vi "PlayChords.vi"() -> (3 "timed out?":bool)   [LabVIEW 2016]
uses:
  <vilib>/Platform/TimedLoop/XDataNode/timing_clust.ctl
  <vilib>/Platform/TimedLoop/XDataNode/nitl_modes.ctl
  <vilib>/Platform/TimedLoop/XDataNode/wakeup.ctl
  <vilib>/sound2/lvsound2.llb/Sound Data Format.ctl
  <vilib>/sound2/lvsound2.llb/Sampling Mode.ctl
  <vilib>/sound2/lvsound2.llb/Sound Output Set Volume (Single).vi
  <vilib>/sound2/lvsound2.llb/Sound Output Write (DBL).vi
  <vilib>/express/express analysis/Spectral/Block/exnSpectralBlock spectral measurements power poly.vi
  <vilib>/express/express analysis/Spectral/Block/exnSpectralBlock spectral measurements power WFM.vi
  <vilib>/platform/TimedLoop/XDataNode/XDataNode.xnode
  <vilib>/express/express analysis/Spectral/XNode/ExpressSpectralMeasurementsBlockNode.xnode
  <vilib>/Platform/TimedLoop/XDataNode/XDNodeRunTimeDep.lvlib
panel:
  out "#Note DiatonicScale":u8
  out "fretPosition":dbl[](array[numeric])
  out "#StringsUsed in Chord":dbl
  out "Power Spectrum":cluster{"f0":dbl, "df":dbl, "magnitude":dbl[]}(graph)
  in  "?":bool
  in  "Volume 2":dbl(knob)=35.90378919003022 scale=20.0..100.0
  in  "strumming rate (in ms)":dbl=10.0
  in  "Upstrum ?":bool
  # "0, 1, 8 -> C mojor chord\n2 -> D major chord\n3 -> E major chord\n4 -> F major chord\n5 -> G major chord\n6 -> A major chord\n7 -> B mojor chord"
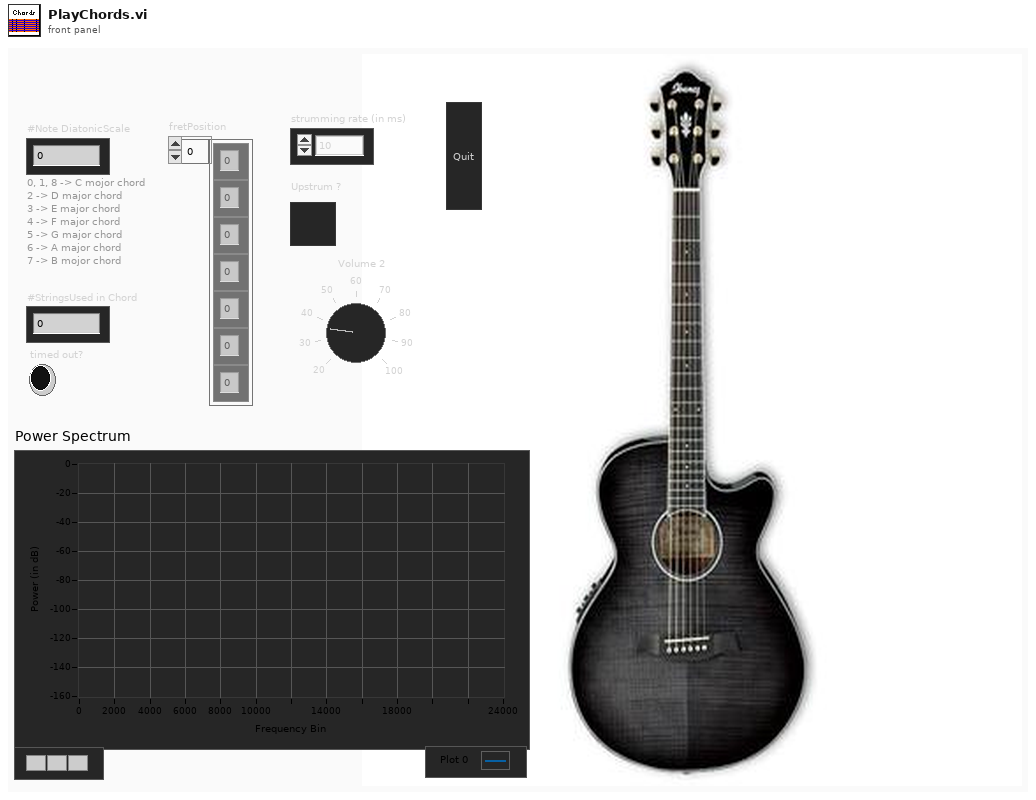
[diagram p1: front panel]
types:
  T1 = typedef "XDNodeRunTimeDep.lvlib/timing_clust.ctl" = cluster{"Expected End [f-1]":u64, "Actual End [f-1]":u64, "Finished Late? [f-1]":bool, "Expected End [i-1]":u64, "Actual End [i-1]":u64, "Finished Late? [i-1]":bool, "Expected Start [i]":u64, "Actual Start [i]":u64, "Expected Start [f]":u64, "Actual Start [f]":u64, "Source Name":string, "Structure Name":string, "Period":i64, "Deadline":i64, "Offset":i64, "Start":i64, "Priority":i32, "Timeout":i32, "Mode":T2, "Wakeup Reason":T3, "Error":errorcluster, "Source Type":string, "Secondary Source Type":string, "Global End Time":u64, "Global Start Time":u64, "Frame Duration":u64, "Iteration Duration":u64, "Assigned CPU":i32, "I/O Scan Engine Mode":u32}
  T2 = typedef "XDNodeRunTimeDep.lvlib/nitl_modes.ctl" = enum32{"No Change", "Process missed periods, maintain original phase", "Discard missed periods, maintain original phase", "Process missed periods, ignore original phase", "Discard missed periods, ignore original phase"}
  T3 = typedef "XDNodeRunTimeDep.lvlib/wakeup.ctl" = enum32{"Normal", "Aborted", "Asynchronous wakeup", "Timing source error", "Timed loop error", "Timeout"}
  T4 = typedef "Sound Data Format.ctl" = cluster{"sample rate (S/s)":dbl, "number of channels":i32, "bits per sample":i32}
  T5 = cluster{"averaging mode":u16, "weighting mode":u16, "number of averages":u32}
  T6 = cluster{"dB On (F)":bool, "unwrap phase (F)":bool, "convert to degree (F)":bool}
  T7 = typedef "Sampling Mode.ctl" = i32
  T8 = typedef "Sound Output Task ID.ctl" = u32
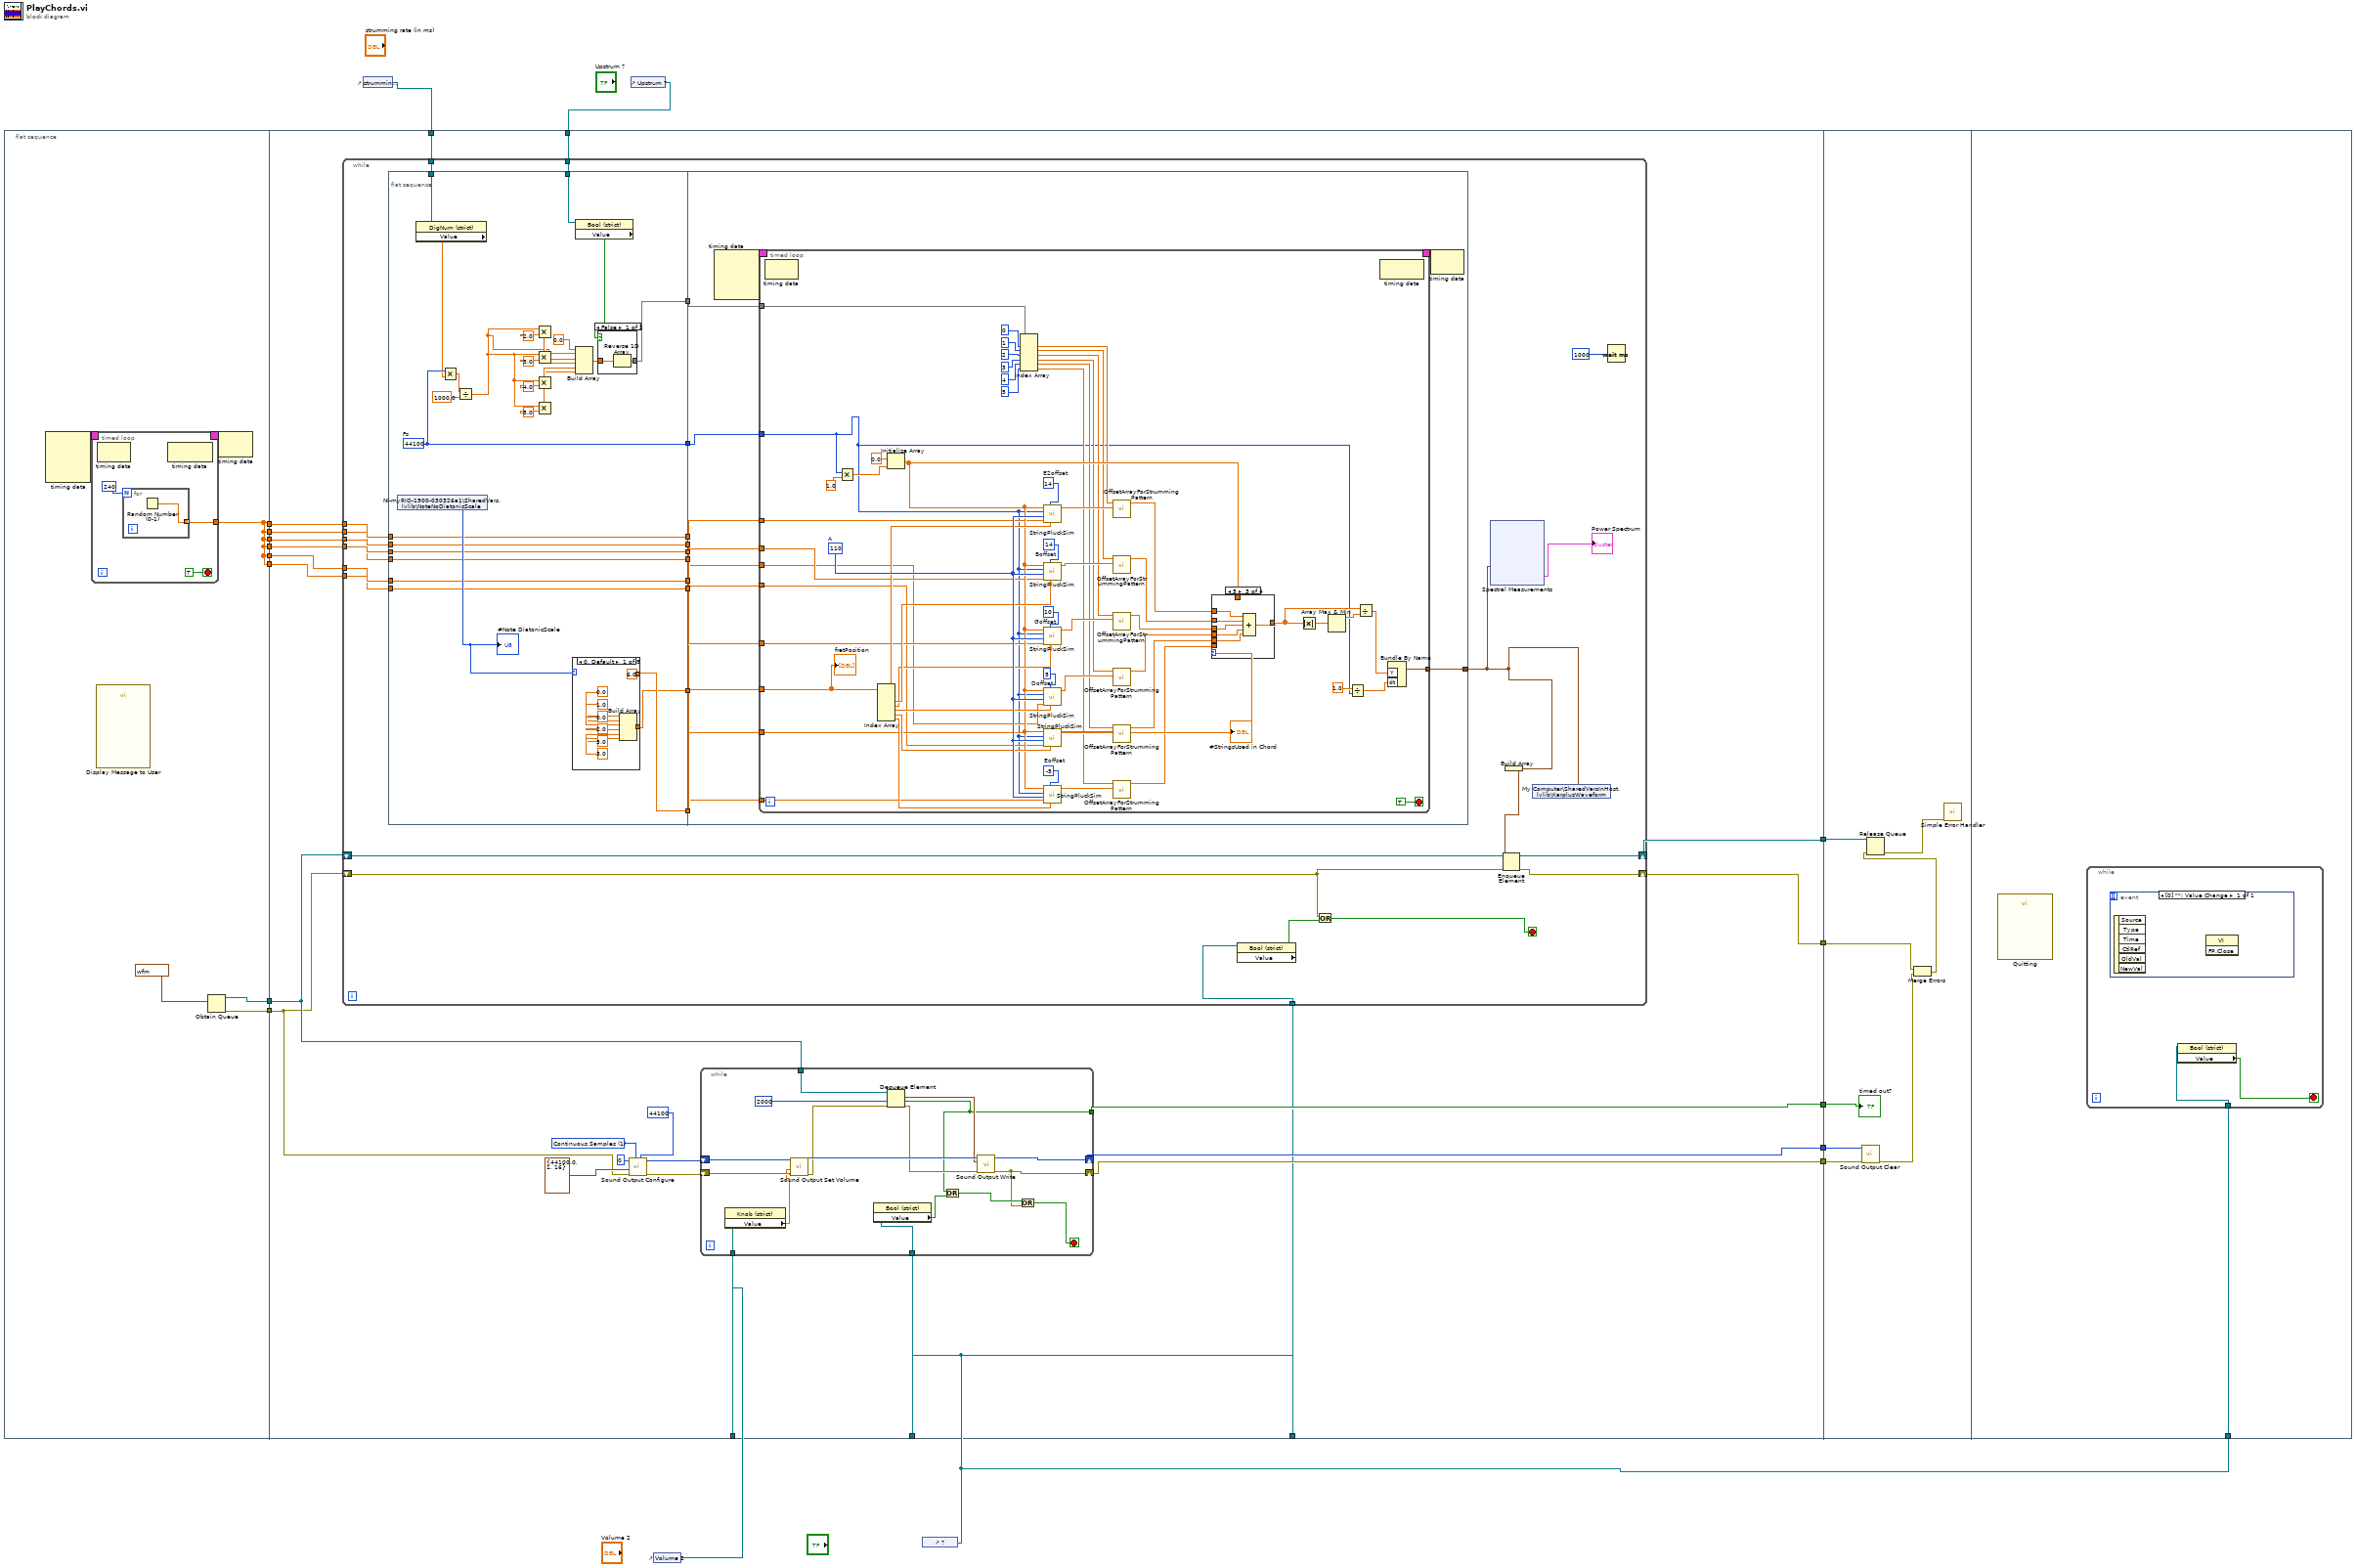
[diagram p0: block diagram]
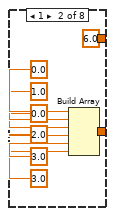
[diagram p3: hidden frame]
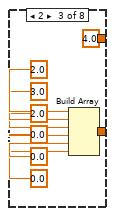
[diagram p4: hidden frame]
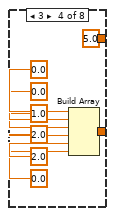
[diagram p5: hidden frame]
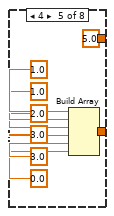
[diagram p6: hidden frame]
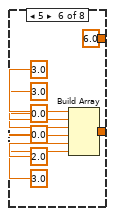
[diagram p7: hidden frame]
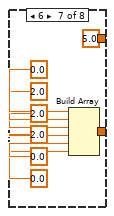
[diagram p8: hidden frame]
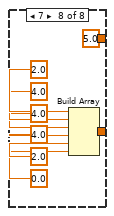
[diagram p9: hidden frame]
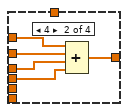
[diagram p11: hidden frame]
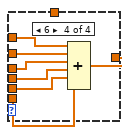
[diagram p12: hidden frame]
diagram:
  n1 = flat-sequence {
    tunnel: [w20] -> w17
    tunnel: [w22] -> w16
    tunnel: [w21] -> w15
    tunnel: [w20] -> w14
    tunnel: [w20] -> w13
    tunnel: [w20] -> w12
    tunnel: [w20] -> w11
    tunnel: [w20] -> w10
    tunnel: w17 -> [w47]
    tunnel: w16 -> [w49]
    tunnel: w15 -> [w48]
    tunnel: w14 -> [w46]
    tunnel: w13 -> [w45]
    tunnel: w12 -> [w44]
    tunnel: w11 -> [w43]
    tunnel: w10 -> [w42]
    tunnel: w3 -> [w41]
    tunnel: w4 -> [w40]
    tunnel: w2 -> [w39]
    tunnel: [w38] -> w9
    tunnel: [w37] -> w8
    tunnel: [w35] -> w7
    tunnel: [w36] -> w6
    tunnel: [w34] -> w5
    tunnel: w1 -> [w33]
    tunnel: w1 -> [w32]
    tunnel: w9 -> [w305]
    tunnel: w8 -> [w304]
    tunnel: w7 -> [w303]
    tunnel: w6 -> [w302]
    tunnel: w5 -> [w301]
    tunnel: w1 -> [w308]
    frame #0 {
      n2 = node-c288() -> (w19:T1)  [unwired: 4 in]
      n3 = timed-loop {
        timing: w19 -> [_]
        timing-out: [_] -> w18
        tunnel: [w25] -> w20
        stop <- TRUE stop-if-true
        n4 = node-c288() -> ()  [unwired: 1 in, 1 out]
        n5 = for {
          N: 240 -> [_]
          tunnel: [w27] -> w25 mode=indexing
          n6 = Random Number (0-1)() -> (number: 0 to 1=w27:dbl)
        }
        n7 = node-c288() -> ()  [unwired: 1 in, 1 out]
      }
      n8 = call "Display Message to User"() -> ()  [unwired: 10 in, 2 out]
      n9 = Obtain Queue(element data type=waveform(dbl)[] [{"t0"=timestamp(3482746353.0334034 s since 1904-01-01), "dt"=4.5351473922902495e-05, "Y"=array[5000 elements]}, {"t0"=timestamp(3482746353.0334034 s since 1904-01-01), "dt"=4.5351473922902495e-05, "Y"=array[5000 elements]}] ("Generated Sound")) -> (queue out=w22:refnum<queue>, error out=w21:errorcluster)  [unwired: 4 in, 1 out]
      n10 = node-c288(w18) -> ()  [unwired: 1 out]
    }
    frame #1 {
      w53 = T7 1 items=["Finite Samples", "Continuous Samples"] ("sample mode")
      n11 = while {
        shift-right: [w82] -> w38
        shift-left: w49 -> [w84]
        shift-right: [w83] -> w37
        shift-left: w48 -> [w80]
        tunnel: w47 -> [w75]
        tunnel: w46 -> [w73]
        tunnel: w45 -> [w71]
        tunnel: w44 -> [w69]
        tunnel: w43 -> [w67]
        tunnel: w42 -> [w65]
        tunnel: w41 -> [w62]
        tunnel: w40 -> [w61]
        tunnel: w32 -> [w59]
        stop <- w81 stop-if-true
        n12 = flat-sequence {
          tunnel: [w120] -> w78
          tunnel: [w119] -> w77
          tunnel: [w118] -> w76
          tunnel: w75 -> [w118]
          tunnel: [w117] -> w74
          tunnel: w73 -> [w117]
          tunnel: [w116] -> w72
          tunnel: w71 -> [w116]
          tunnel: [w115] -> w70
          tunnel: w69 -> [w115]
          tunnel: [w114] -> w68
          tunnel: w67 -> [w114]
          tunnel: [w113] -> w66
          tunnel: w65 -> [w113]
          tunnel: [w102] -> w64
          tunnel: [w101] -> w63
          tunnel: w62 -> [w97]
          tunnel: w61 -> [w95]
          tunnel: [w201] -> w56
          tunnel: w78 -> [w200]
          tunnel: w77 -> [w199]
          tunnel: w76 -> [w198]
          tunnel: w74 -> [w197]
          tunnel: w72 -> [w196]
          tunnel: w70 -> [w195]
          tunnel: w68 -> [w194]
          tunnel: w66 -> [w193]
          tunnel: w64 -> [w192]
          tunnel: w63 -> [w191]
          frame #0 {
            w101 = 44100  # Fs
            n13 = shared-variable "NI-myRIO-1900-030326a1\\SharedVars.lvlib\\NoteNoDiatonicScale"() -> (w121:u8)  [unwired: 1 in, 1 out]
            "#Note DiatonicScale" <- w121
            n14 = property class="DigNum (strict)"(reference=w97) -> ("Value"=w96:dbl)  [unwired: 1 in, 2 out]
            n15 = Multiply(x=w101, y=w96) -> (x*y=w100:dbl)
            n16 = Divide(x=w100, y=1000.0) -> (x/y=w98:dbl)
            n17 = Multiply(x=w98, y=2.0) -> (x*y=w107:dbl)
            n18 = Multiply(x=w98, y=3.0) -> (x*y=w106:dbl)
            n19 = Multiply(x=w98, y=4.0) -> (x*y=w105:dbl)
            n20 = Multiply(x=w98, y=5.0) -> (x*y=w104:dbl)
            n21 = case shown="0, Default" w121 {
              tunnel: [6.0 ("element") 6.0 ("element") 4.0 ("element") 5.0 ("element") 5.0 ("element") 6.0 ("element") 5.0 ("element") 5.0 ("element")] -> w120
              tunnel: [w126 w134 w142 w150 w158 w166 w174 w182] -> w119
              frame 0, Default {
                n22 = Build Array(0.0 ("element"), 1.0 ("element"), 0.0 ("element"), 2.0 ("element"), 3.0 ("element"), 3.0 ("element")) -> (w126:dbl[])
              }
              frame 1 {
                n23 = Build Array(0.0 ("element"), 1.0 ("element"), 0.0 ("element"), 2.0 ("element"), 3.0 ("element"), 3.0 ("element")) -> (w134:dbl[])
              }
              frame 2 {
                n24 = Build Array(2.0 ("element"), 3.0 ("element"), 2.0 ("element"), 0.0 ("element"), 0.0 ("element"), 0.0 ("element")) -> (w142:dbl[])
              }
              frame 3 {
                n25 = Build Array(0.0 ("element"), 0.0 ("element"), 1.0 ("element"), 2.0 ("element"), 2.0 ("element"), 0.0 ("element")) -> (w150:dbl[])
              }
              frame 4 {
                n26 = Build Array(1.0 ("element"), 1.0 ("element"), 2.0 ("element"), 3.0 ("element"), 3.0 ("element"), 0.0 ("element")) -> (w158:dbl[])
              }
              frame 5 {
                n27 = Build Array(3.0 ("element"), 3.0 ("element"), 0.0 ("element"), 0.0 ("element"), 2.0 ("element"), 3.0 ("element")) -> (w166:dbl[])
              }
              frame 6 {
                n28 = Build Array(0.0 ("element"), 2.0 ("element"), 2.0 ("element"), 2.0 ("element"), 0.0 ("element"), 0.0 ("element")) -> (w174:dbl[])
              }
              frame 7 {
                n29 = Build Array(2.0 ("element"), 4.0 ("element"), 4.0 ("element"), 4.0 ("element"), 2.0 ("element"), 0.0 ("element")) -> (w182:dbl[])
              }
            }
            n30 = property class="Bool (strict)"(reference=w95) -> ("Value"=w94:bool)  [unwired: 1 in, 2 out]
            n31 = Build Array(0.0 ("element"), w98, w107, w106, w105, w104) -> (w103:dbl[])
            n32 = case shown="False" w94 {
              tunnel: w103 -> [w123 w124]
              tunnel: [w122 w124] -> w102
              frame False {
                n33 = Reverse 1D Array(array=w123) -> (reversed array=w122:dbl[])
              }
              frame True {
              }
            }
          }
          frame #1 {
            n34 = node-c288() -> (w190:T1)  [unwired: 4 in]
            n35 = timed-loop {
              timing: w190 -> [_]
              timing-out: [_] -> w189
              tunnel: [w238] -> w201
              tunnel: w200 -> [w236]
              tunnel: w199 -> [w235]
              tunnel: w198 -> [w234]
              tunnel: w197 -> [w233]
              tunnel: w196 -> [w232]
              tunnel: w195 -> [w231]
              tunnel: w194 -> [w230]
              tunnel: w193 -> [w229]
              tunnel: w192 -> [w217]
              tunnel: w191 -> [w203]
              stop <- TRUE stop-if-true
              w247 = 5  # Doffset
              w246 = 10  # Goffset
              w249 = 14  # Boffset
              w250 = 14  # E2offset
              w248 = -5  # Eoffset
              w257 = 110  # A
              n36 = node-c288() -> ()  [unwired: 1 in, 1 out]
              n37 = Multiply(x=w203, y=1.0 ("element")) -> (x*y=w259:dbl)
              n38 = Index Array(array=w235) -> (element #1=w256:dbl, element #2=w255:dbl, element #3=w254:dbl, element #4=w253:dbl, element #5=w252:dbl, element #6=w251:dbl)  [unwired: 6 in]
              n39 = Initialize Array(0.0 ("element"), w259) -> (w245:dbl[])
              n40 = Index Array(array=w217, index #1=0 ("index"), index #2=1 ("index"), index #3=2 ("index"), index #4=3 ("index"), index #5=4 ("index"), index #6=5 ("index")) -> (element #1=w210:dbl, element #2=w209:dbl, element #3=w208:dbl, element #4=w207:dbl, element #5=w206:dbl, element #6=w205:dbl)
              n41 = call "StringPluckSim.vi"("fretPos"=w256, "offset"=w250, "Initial Random Array"=w234, "A"=w257, "Fs"=w203, "InitialArray"=w245) -> ("PluckedStringOut"=w228:dbl[])  [unwired: 5 in]
              n42 = call "StringPluckSim.vi"("fretPos"=w255, "offset"=w249, "Initial Random Array"=w233, "A"=w257, "Fs"=w203, "InitialArray"=w245) -> ("PluckedStringOut"=w226:dbl[])  [unwired: 5 in]
              n43 = call "StringPluckSim.vi"("fretPos"=w254, "offset"=w246, "Initial Random Array"=w232, "A"=w257, "Fs"=w203, "InitialArray"=w245) -> ("PluckedStringOut"=w224:dbl[])  [unwired: 5 in]
              n44 = call "StringPluckSim.vi"("fretPos"=w253, "offset"=w247, "Initial Random Array"=w231, "A"=w257, "Fs"=w203, "InitialArray"=w245) -> ("PluckedStringOut"=w223:dbl[])  [unwired: 5 in]
              n45 = call "StringPluckSim.vi"("fretPos"=w252, "Initial Random Array"=w230, "A"=w257, "Fs"=w203, "InitialArray"=w245) -> ("PluckedStringOut"=w221:dbl[])  [unwired: 6 in]
              n46 = call "StringPluckSim.vi"("fretPos"=w251, "offset"=w248, "Initial Random Array"=w229, "A"=w257, "Fs"=w203, "InitialArray"=w245) -> ("PluckedStringOut"=w219:dbl[])  [unwired: 5 in]
              n47 = call "OffsetArrayForStrummingPattern.vi"("input array"=w228, "offset"=w210) -> ("Array"=w227:dbl[])  [unwired: 9 in]
              n48 = call "OffsetArrayForStrummingPattern.vi"("input array"=w226, "offset"=w209) -> ("Array"=w225:dbl[])  [unwired: 9 in]
              n49 = call "OffsetArrayForStrummingPattern.vi"("input array"=w224, "offset"=w208) -> ("Array"=w204:dbl[])  [unwired: 9 in]
              n50 = call "OffsetArrayForStrummingPattern.vi"("input array"=w223, "offset"=w207) -> ("Array"=w222:dbl[])  [unwired: 9 in]
              n51 = call "OffsetArrayForStrummingPattern.vi"("input array"=w221, "offset"=w206) -> ("Array"=w220:dbl[])  [unwired: 9 in]
              n52 = call "OffsetArrayForStrummingPattern.vi"("input array"=w219, "offset"=w205) -> ("Array"=w218:dbl[])  [unwired: 9 in]
              n53 = case shown="5" w236 {
                tunnel: w245 -> [w260 _ _ _]
                tunnel: [w260 w261 w267 w274] -> w243
                tunnel: w227 -> [_ w265 w271 w278]
                tunnel: w225 -> [_ w264 w270 w277]
                tunnel: w204 -> [_ w263 w269 w276]
                tunnel: w222 -> [_ w262 w268 w275]
                tunnel: w220 -> [_ _ w266 w273]
                tunnel: w218 -> [_ _ _ w272]
                frame 0, Default {
                }
                frame 4 {
                  n54 = Compound Arithmetic op=ADD(w265, w264, w263, w262) -> (w261:dbl[])
                }
                frame 5 {
                  n55 = Compound Arithmetic op=ADD(w271, w270, w269, w268, w266) -> (w267:dbl[])
                }
                frame 6 {
                  n56 = Compound Arithmetic op=ADD(w278, w277, w276, w275, w273, w272) -> (w274:dbl[])
                }
              }
              n57 = Absolute Value(x=w243) -> (abs(x)=w244:dbl[])
              n58 = Array Max & Min(array=w244) -> (max value=w242:dbl)  [unwired: 3 out]
              n59 = Divide(x=1.0, y=w203) -> (x/y=w239:dbl)
              n60 = Divide(x=w243, y=w242) -> (x/y=w241:dbl[])
              n61 = node-c288() -> ()  [unwired: 1 in, 1 out]
              n62 = Bundle By Name("Y"=w241, "dt"=w239) -> (w238:waveform(dbl))  [unwired: 1 in]
              "fretPosition" <- w235
              "#StringsUsed in Chord" <- w236
            }
            n63 = node-c288(w189) -> ()  [unwired: 1 out]
          }
        }
        n64 = property class="Bool (strict)"(reference=w59) -> ("Value"=w58:bool)  [unwired: 1 in, 2 out]
        n65 = Or(x=w80, y=w58) -> (x .or. y?=w81:bool)
        n66 = xnode "Spectral Measurements"("Signals"=w56) -> ("Power Spectrum"=→"Power Spectrum":cluster{"f0":dbl, "df":dbl, "magnitude":dbl[]})  [unwired: 1 in, 1 out]
        n67 = Build Array(w56) -> (w60:waveform(dbl)[])
        n68 = Enqueue Element(queue=w84, element=w60, error in (no error)=w80) -> (queue out=w82:refnum<queue>, error out=w83:errorcluster)  [unwired: 1 in, 1 out]
        n69 = shared-variable "My Computer\\SharedVarsInHost.lvlib\\KarplusWaveform"(w56) -> ()  [unwired: 1 in, 1 out]
        n70 = Wait (ms)(milliseconds to wait=u32 1000) -> ()  [unwired: 1 out]
      }
      n71 = call <vilib>:"Sound Output Configure.vi"("number of samples/ch"=44100, "sample mode"=w53, "error in (no error)"=w48, "sound format"=T4 {"sample rate (S/s)"=44100.0, "number of channels"=1, "bits per sample"=16}, "device ID"=u32 0) -> ("error out"=w51:errorcluster, "task ID"=w52:T8)  [unwired: 5 in]
      n72 = while {
        shift-right: [w296] -> w36
        shift-left: w52 -> [w299]
        shift-right: [w289] -> w35
        shift-left: w51 -> [w298]
        tunnel: w49 -> [w295]
        tunnel: w39 -> [w287]
        tunnel: [w285] -> w34
        tunnel: w33 -> [w284]
        stop <- w288 stop-if-true
        n73 = property class="Knob (strict)"(reference=w287) -> ("Value"=w286:dbl)  [unwired: 1 in, 2 out]
        n74 = call-poly <vilib>:"Sound Output Set Volume.vi"("error in (no error)"=w298, "volume"=w286, "task ID"=w299) -> ("error out"=w294:errorcluster, "task ID out"=w297:T8)  [unwired: 7 in]
        n75 = property class="Bool (strict)"(reference=w284) -> ("Value"=w283:bool)  [unwired: 1 in, 2 out]
        n76 = Dequeue Element(queue=w295, timeout in ms (-1)=2000, error in (no error)=w294) -> (element=w293:waveform(dbl)[], timed out?=w285:bool, error out=w291:errorcluster)  [unwired: 1 out]
        n77 = Or(x=w285, y=w283) -> (x .or. y?=w290:bool)
        n78 = call-poly <vilib>:"Sound Output Write.vi"("error in (no error)"=w291, "data"=w293, "task ID"=w297) -> ("error out"=w289:errorcluster, "task ID out"=w296:T8)  [unwired: 7 in]
        n79 = Or(x=w290, y=w289) -> (x .or. y?=w288:bool)
      }
    }
    frame #2 {
      n80 = call <vilib>:"Sound Output Clear.vi"("error in (no error)"=w303, "task ID"=w302) -> ("error out"=w300:errorcluster)  [unwired: 9 in]
      n81 = Merge Errors(w304, w300) -> (w307:errorcluster)
      n82 = Release Queue(queue=w305, error in (no error)=w307) -> (error out=w306:errorcluster)  [unwired: 1 in, 2 out]
      n83 = call <vilib>:"Simple Error Handler.vi"("error in (no error)"=w306) -> ()  [unwired: 4 in, 5 out]
      "timed out?" <- w301
    }
    frame #3 {
      n84 = call "Quitting"() -> ()  [unwired: 10 in, 2 out]
      n85 = while {
        tunnel: w308 -> [w310]
        stop <- w309 stop-if-true
        n86 = event shown="[0] \"\": Value Change" {
          selector: _ -> [_]
          dyn-events: _ -> [_]
          timeout: _ -> [_]
          event Value Change {
            n87 = event-data() -> ()  [unwired: 1 in, 6 out]
            n88 = invoke class="VI" method="FP.Close"() -> ()  [unwired: 3 in, 3 out]
          }
        }
        n89 = property class="Bool (strict)"(reference=w310) -> ("Value"=w309:bool)  [unwired: 1 in, 2 out]
      }
    }
  }
  n90 = control-ref of="strumming rate (in ms)"() -> (w3:refnum<vi>)
  n91 = control-ref of="Upstrum ?"() -> (w4:refnum<vi>)
  n92 = control-ref of="Volume 2"() -> (w2:refnum<vi>)
  n93 = control-ref of="?"() -> (w1:refnum<vi>)
